vi "Delete from Array (Value).vi"(8 "error in (no error)":errorcluster, 9 "index":i32, 11 "JSON Value in":refnum<class "JSON Value.lvclass">) -> (0 "error out":errorcluster, 1 "JSON Value out":refnum<class "JSON Value.lvclass">, 3 "JSON Value out":refnum<class "JSON Value.lvclass">)   [LabVIEW 2016, in "JSON Value.lvclass"]
doc: "Deletes an element or subarray from a JSON array of length elements starting at index. Returns the edited array in array w/ subset deleted and the deleted element or subarray in deleted portion."
uses:
  JSON Value.lvclass
  JSON Value.lvclass/JSON Value.ctl
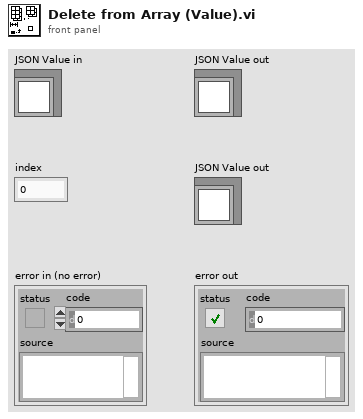
[diagram p1: front panel]
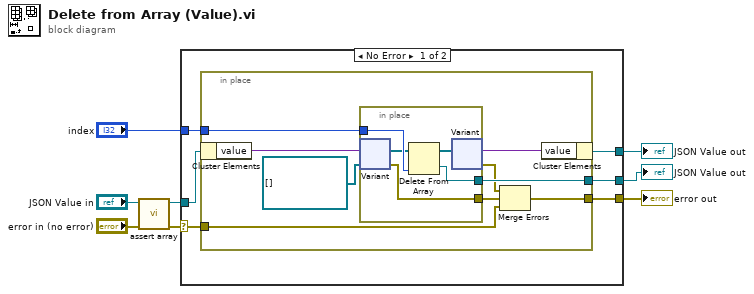
[diagram p0: block diagram]
diagram:
  n1 = call "assert array.vi"("error in (no error)"="error in (no error)", "JSON Value in"="JSON Value in") -> ("error out"=w3:errorcluster, "JSON Value out"=w4:refnum<class "JSON Value.lvclass">)  [unwired: 8 in]
  n2 = case shown="No Error" w3 {
    selector: w3 -> [w10 w29]
    tunnel: "index" -> [w14 _]
    tunnel: [w13 w30] -> w6
    tunnel: [w12 _] -> w5
    tunnel: w4 -> [w11 w30]
    tunnel: [w9 w29] -> w1
    frame No Error {
      n3 = in-place {
        in-place-border: w14 -> [w23]
        in-place-border: [w22] -> w12
        in-place-border: w10 -> [w16]
        in-place-border: [w15] -> w9
        n4 = in-place-cluster #1(w11) -> ("value"=w21:variant)
        n5 = in-place {
          in-place-border: w23 -> [w28]
          in-place-border: [w27] -> w22
          in-place-border: [w24] -> w18
          n6 = in-place-variant #2(w21, refnum<class "JSON Value.lvclass">[] [] ("LVJSON.lvlib:JSON Array In")) -> (w26:refnum<class "JSON Value.lvclass">[], w24:errorcluster)
          n7 = Delete From Array(array=w26, index=w28) -> (deleted portion=w27:refnum<class "JSON Value.lvclass">, array with subset deleted=w25:refnum<class "JSON Value.lvclass">[])  [unwired: 1 in]
          n8 = in-place-variant #2(w25) -> (w19:variant, w17:errorcluster)
        }
        n9 = Merge Errors(w17, w18, w16) -> (w15:errorcluster)
        n10 = in-place-cluster #1("value"=w19) -> (w13:refnum<class "JSON Value.lvclass">)
      }
    }
    frame Error {
    }
  }
  "JSON Value out" <- w5
  "JSON Value out" <- w6
  "error out" <- w1
